vi "Configure Protection Disconnect.vi"(7 "Disconnect Method (0: High Impedance)":u16(ring) items=["High Impedance", "Low Impedance"], 8 "error in (no error)":errorcluster, 11 "VISA resource name":refnum<visa-resource-name>) -> (0 "error out":errorcluster, 3 "VISA resource name out":refnum<visa-resource-name>)   [LabVIEW 2019, in "Agilent N7976A.lvlib"]
doc: "Configures the disconnect method for protections."
uses:
  <instrlib>/Agilent N7976A/Agilent N7976A.lvlib
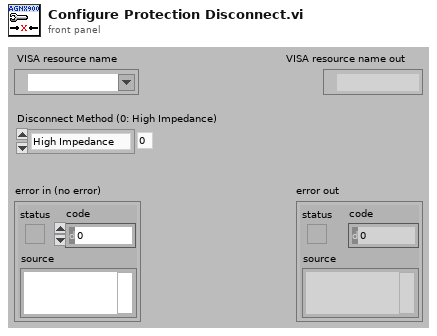
[diagram p1: front panel]
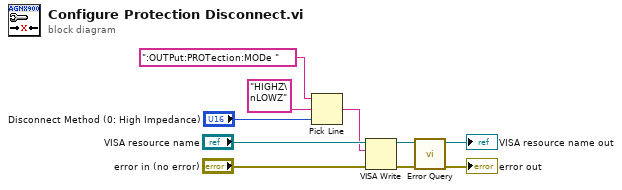
[diagram p0: block diagram]
diagram:
  n1 = Pick Line(string ("")=":OUTPut:PROTection:MODe " ("format string"), multi-line string="HIGHZ\nLOWZ", line index="Disconnect Method (0: High Impedance)") -> (output string=w2:string)
  n2 = VISA Write(VISA resource name="VISA resource name", write buffer=w2, error in (no error)="error in (no error)") -> (VISA resource name out=w7:refnum<visa-resource-name>, error out=w8:errorcluster)  [unwired: 1 out]
  n3 = call <instrlib>:"Error Query.vi"("error in (no error)"=w8, "VISA resource name"=w7) -> ("error out"=→"error out":errorcluster, "VISA resource name out"=→"VISA resource name out":refnum<visa-resource-name>)  [unwired: 6 in, 2 out]
